vi "oax_Play Sound.vi"(7 "sound format":T1={"sample rate (S/s)"=22050.0, "number of channels"=2, "bits per sample"=16}, 8 "error in (no error)":errorcluster, 11 "waveform to play":waveform(dbl)={"t0"=timestamp(0 s since 1904-01-01), "dt"=0.0, "Y"=[]}) -> (0 "error out":errorcluster)   [LabVIEW 2017]
doc: "Plays the waveform through the sound card."
uses:
  <vilib>/sound2/lvsound2.llb/Sound Data Format.ctl
  <vilib>/sound2/lvsound2.llb/Sampling Mode.ctl
  <vilib>/sound2/lvsound2.llb/Sound Output Write (DBL Single).vi
  <vilib>/Waveform/WDTOps.llb/WDT Waveform Duration DBL.vi
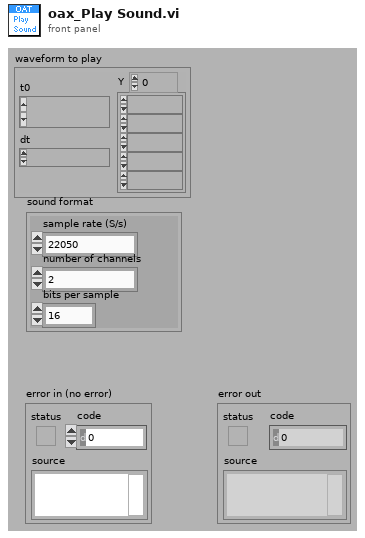
[diagram p1: front panel]
types:
  T1 = typedef "Sound Data Format.ctl" = cluster{"sample rate (S/s)":dbl, "number of channels":i32, "bits per sample":i32}
  T2 = typedef "Sampling Mode.ctl" = i32
  T3 = typedef "Sound Output Task ID.ctl" = u32
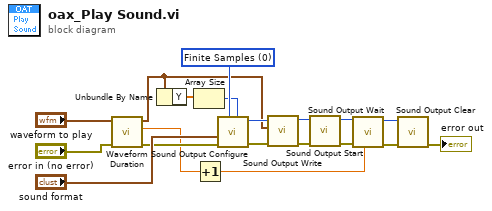
[diagram p0: block diagram]
diagram:
  w6 = T2 0 items=["Finite Samples", "Continuous Samples"] ("sample mode")
  n1 = call-poly <vilib>:"Waveform Duration.vi"("error in (no error)"="error in (no error)", "waveform in"="waveform to play") -> ("error out"=w8:errorcluster, "duration"=w2:dbl, "waveform out"=w5:waveform(dbl))  [unwired: 7 in]
  n2 = Unbundle By Name(w5) -> ("Y"=w4:dbl[])
  n3 = Array Size(array=w4) -> (size(s)=w3:i32)
  n4 = Increment(x=w2) -> (x+1=w1:dbl)
  n5 = call <vilib>:"Sound Output Configure.vi"("number of samples/ch"=w3, "sample mode"=w6, "error in (no error)"=w8, "sound format"="sound format") -> ("error out"=w19:errorcluster, "task ID"=w18:T3)  [unwired: 6 in]
  n6 = call-poly <vilib>:"Sound Output Write.vi"("error in (no error)"=w19, "data"=w5, "task ID"=w18) -> ("error out"=w17:errorcluster, "task ID out"=w16:T3)  [unwired: 7 in]
  n7 = call <vilib>:"Sound Output Start.vi"("error in (no error)"=w17, "task ID"=w16) -> ("error out"=w15:errorcluster, "task ID out"=w14:T3)  [unwired: 8 in]
  n8 = call <vilib>:"Sound Output Wait.vi"("timeout (sec)"=w1, "error in (no error)"=w15, "task ID"=w14) -> ("error out"=w13:errorcluster, "task ID out"=w12:T3)  [unwired: 7 in]
  n9 = call <vilib>:"Sound Output Clear.vi"("error in (no error)"=w13, "task ID"=w12) -> ("error out"=→"error out":errorcluster)  [unwired: 9 in]
